vi "Determine Decimation Rate.vi"(10 "Rate (Hz)":dbl, 11 "J1939 Settings":T1={"XNET Database"="", "XNET Cluster"="", "CAN Port"="", "Baud rate [Bd]"=0, "Termination"=0, "Incoming Rate"=0, "Outcoming Rate"=0, "Write Decimation"=1} {"Termination" items=["Off", "On"]}) -> (2 "Outgoing Decimation":u32, 3 "Incoming Decimation":u32)   [LabVIEW 2013, in "J1939 Addon Engine.lvlib"]
uses:
  J1939 Addon Engine.lvlib
  Shared/Types/XNET Settings.ctl
  Shared/J1939 Addon Shared.lvlib
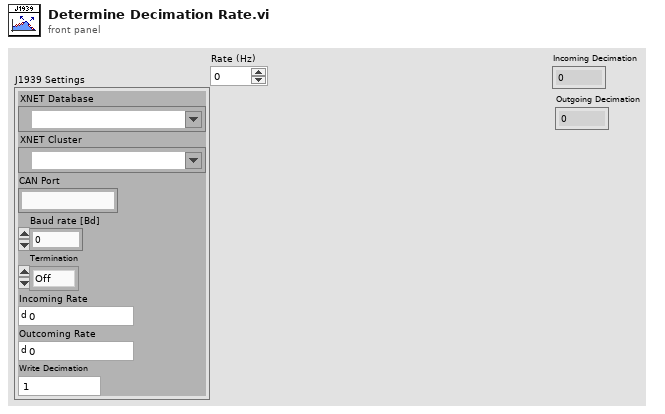
[diagram p1: front panel]
types:
  T1 = typedef "J1939 Addon Shared.lvlib/XNET Settings.ctl" = cluster{"XNET Database":refnum<k21>, "XNET Cluster":refnum<k21>, "CAN Port":string, "Baud rate [Bd]":u32, "Termination":u32, "Incoming Rate":u32, "Outcoming Rate":u32, "Write Decimation":u32}
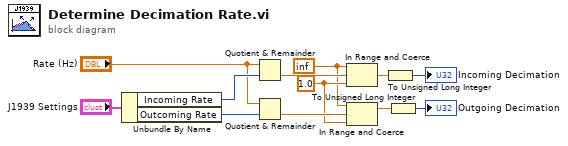
[diagram p0: block diagram]
diagram:
  w3 = inf
  w5 = 1.0 ("lower limit")
  n1 = Unbundle By Name("J1939 Settings") -> ("Incoming Rate"=w11:u32, "Outcoming Rate"=w9:u32)
  n2 = Quotient & Remainder(x="Rate (Hz)", y=w11) -> (floor(x/y)=w8:dbl)  [unwired: 1 out]
  n3 = Quotient & Remainder(x="Rate (Hz)", y=w9) -> (floor(x/y)=w6:dbl)  [unwired: 1 out]
  n4 = In Range and Coerce(upper limit=w3, x=w8, lower limit=w5) -> (coerced(x)=w7:dbl)  [unwired: 1 out]
  n5 = In Range and Coerce(upper limit=w3, x=w6, lower limit=w5) -> (coerced(x)=w4:dbl)  [unwired: 1 out]
  n6 = To Unsigned Long Integer(number=w7) -> (unsigned 32bit integer=→"Incoming Decimation":u32)
  n7 = To Unsigned Long Integer(number=w4) -> (unsigned 32bit integer=→"Outgoing Decimation":u32)
